vi "Automatic Frequency Linearization.vi"() -> ()   [LabVIEW 2014]
panel:
  out "Triangular skewtri generated from min factor":dbl[](graph)
  in  "Sample /Modulation Frequency":enum32{"40MHz/32KHz", "30MHz/24Khz"}(radio)=enum."30MHz/24Khz"
  in  "Scaling factor":dbl=1.0
  out "Rising Min Factor":dbl
  out "Falling Min Factor":dbl
  out "Rising Min DevStd%":dbl
  out "Falling Min DevStd%":dbl
  out "Fine?":bool
  out "Ok?":bool
  in  "#MeanMeasuraments":i32=50
  in  "StopValue":dbl=0.2
  in  "stop":bool
  out "Mean  FREQUENCY Curve Falling":dbl[](graph)
  out "Mean FREQUENCY Curve Rising":dbl[](graph)
  out "Current Skew Tri":dbl[](graph)
  out "Current Mul factor":dbl
  out "Current iteration (Countdown)":dbl
  out "Rising<= 1%":bool
  out "Falling<= 1%":bool
  in  "DeltaFactor":dbl=0.01
  in  "Initial Factor Mul":dbl=0.35
  out "2) Rising StdDev % Graph":cluster{dbl[], dbl[]}(graph)
  out "1) Falling StdDev % Graph":cluster{dbl[], dbl[]}(graph)
  out "2) Rising Std Dev %":dbl
  out "1) Falling Std Dev %":dbl
  out "2) Rising Signal (Last)":dbl[](graph)
  out "1) Falling Signal (Last)":dbl[](graph)
  in  "#LinMesuraments":i32=20
  # "OFFLINE SETUP"
  # "CURRENT ITERATION"
  # "Fattore moltiplicativo"
  # "Numero di misure su cui calcolare la curva delle frequenze medie con triangolo dritto"
  # "Numero di misurazioni\n su cui mediare durante la\nlinearizzazione"
  # "Optimal Factor Rising: 0.33    with Falling curve: 0.294"
  # "Optimal Factor Falling: 0.22/0.23"
  # "Fattore moltiplicativo\nIniziale"
  # "Passo del fattore\nmoltiplicativo"
  # "Fattore moltiplicativo\nFinale"
  # "%"
  # "%"
  # "FINAL RESULTS"
  # "Andamento della deviazione standard percentuale in funzione del fattore moltiplicativo"
  # "%"
  # "%"
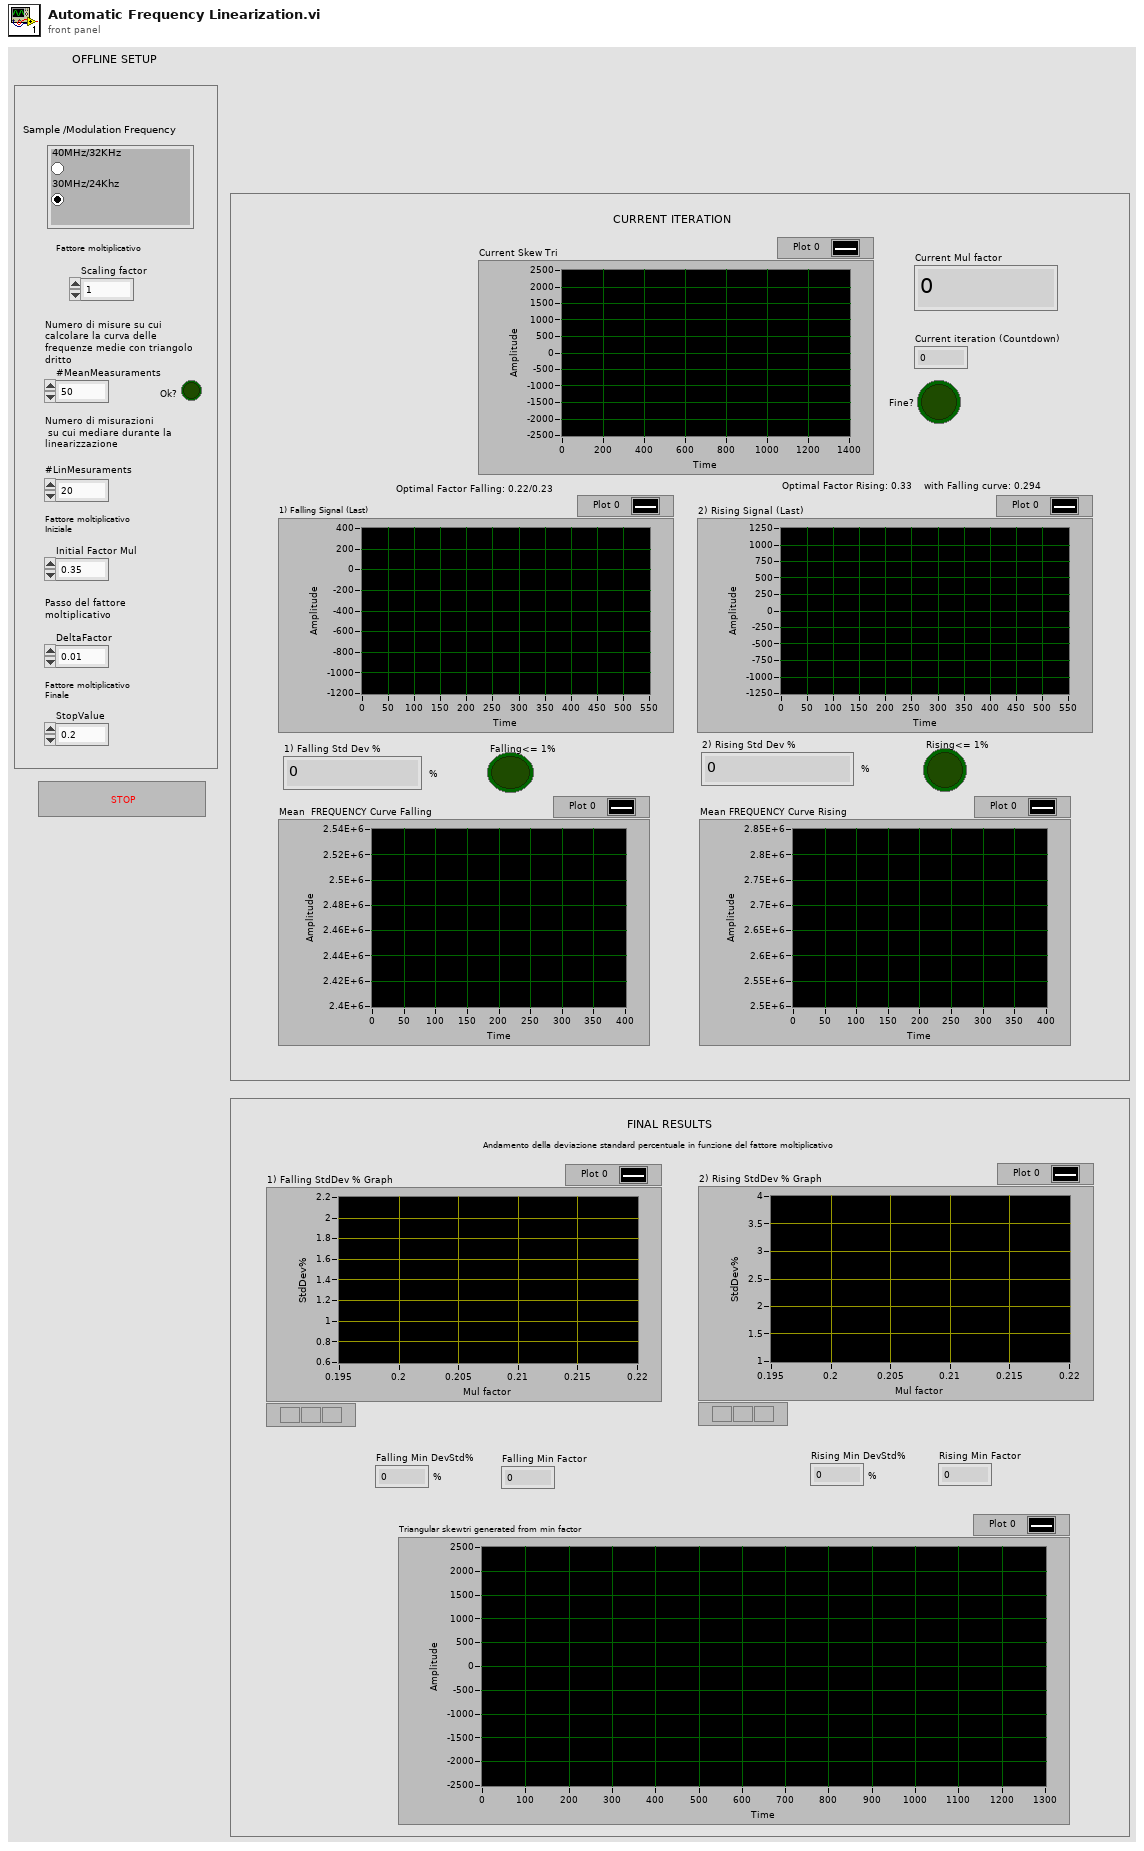
[diagram p1: front panel]
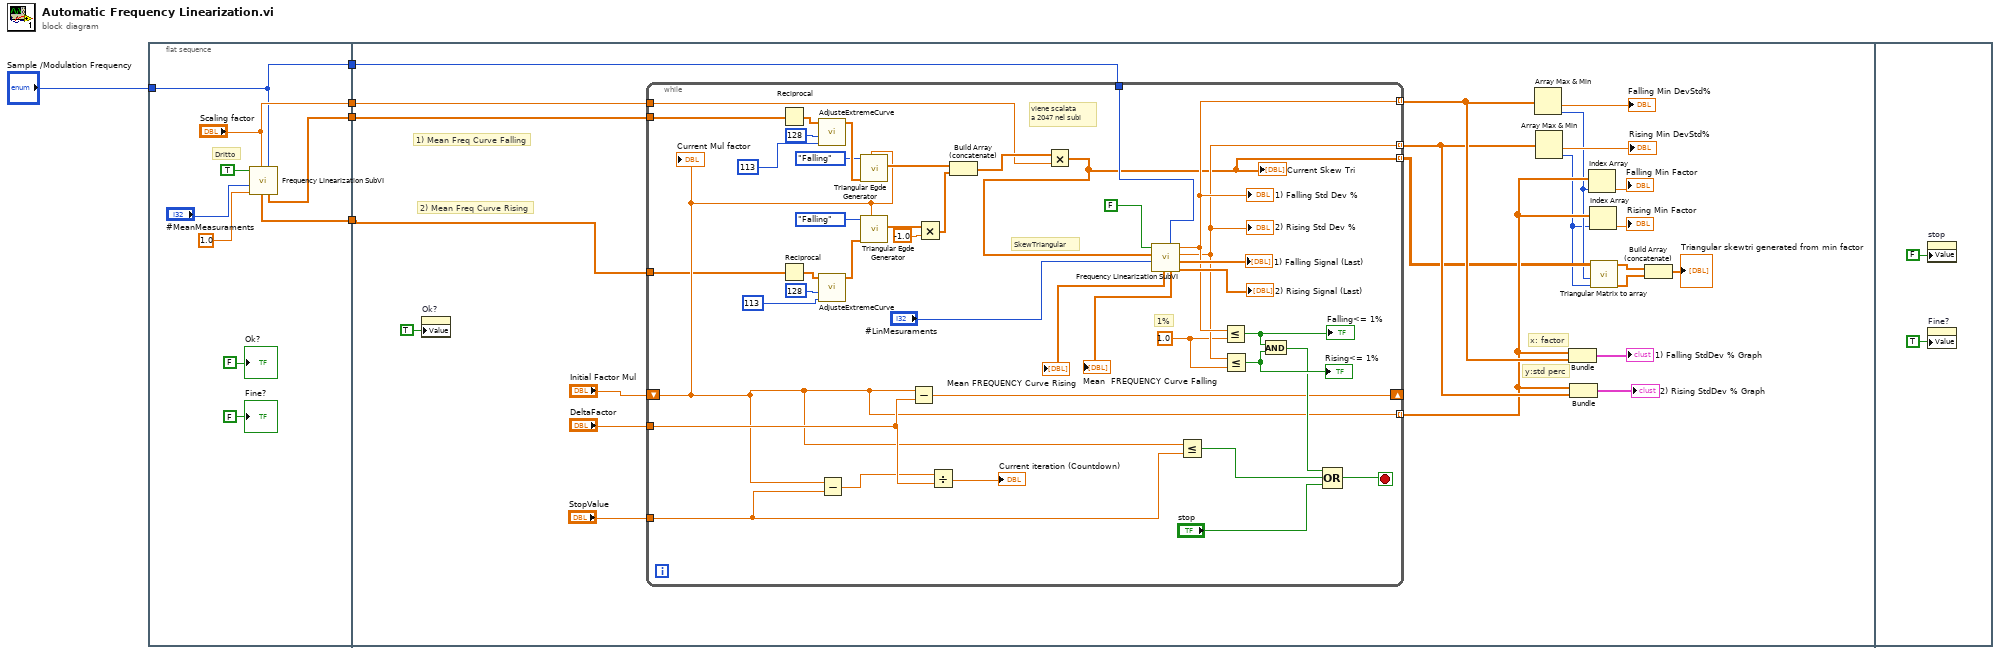
[diagram p0: block diagram]
diagram:
  n1 = flat-sequence {
    tunnel: [w12] -> w5
    tunnel: [w11] -> w4
    tunnel: ["Scaling factor"] -> w3
    tunnel: "Sample /Modulation Frequency" -> [w6]
    tunnel: [w6] -> w1
    tunnel: w5 -> [w23]
    tunnel: w4 -> [w24]
    tunnel: w3 -> [w22]
    tunnel: w1 -> [w21]
    frame #0 {
      # "Dritto"
      n2 = call "Frequency Linearization SubVI.vi"("Sample /Modulation Frequency"=w6, "Scaling factor"="Scaling factor", "Scale factor"=1.0, "#Medie"="#MeanMeasuraments", "Triangolo dritto"=TRUE) -> ("Last Mean Freq Curve Falling"=w12:dbl[], "Last Mean Freq Curve Rising"=w11:dbl[])  [unwired: 1 in, 4 out]
      "Ok?" <- FALSE ("Ok?")
      "Fine?" <- FALSE ("Ok?")
    }
    frame #1 {
      # "2) Mean Freq Curve Rising"
      # "1) Mean Freq Curve Falling"
      # "y:std perc"
      # "x: factor"
      n3 = property on="Ok?" class="Bool (strict)"("Value"=TRUE ("Ok?")) -> ()  [unwired: 2 in, 2 out]
      n4 = while {
        tunnel: [w74] -> w31 mode=indexing
        tunnel: [w73] -> w28 mode=indexing
        shift-right: [w49] -> _
        shift-left: "Initial Factor Mul" -> [w46]
        tunnel: "DeltaFactor" -> [w47]
        tunnel: w23 -> [w41]
        tunnel: w24 -> [w40]
        tunnel: [w46] -> w27 mode=indexing
        tunnel: "StopValue" -> [w45]
        tunnel: w22 -> [w42]
        tunnel: w21 -> [w39]
        tunnel: [w38] -> w20 mode=indexing
        stop <- w52 stop-if-true
        w72 = 1.0 ("y")
        # "viene scalata \na 2047 nel subi"
        # "SkewTriangular"
        # "1%"
        n5 = Reciprocal(x=w41) -> (1/x=w59:dbl[])
        n6 = Reciprocal(x=w40) -> (1/x=w70:dbl[])
        n7 = call "AdjusteExtremeCurve.vi"("Init Bins Discarded"=u32 113, "FFT Size Window"=128, "Freq sample"=w59) -> ("Extended Freq Sample"=w63:dbl[])  [unwired: 8 in]
        n8 = call "AdjusteExtremeCurve.vi"("Init Bins Discarded"=u32 113, "FFT Size Window"=128, "Freq sample"=w70) -> ("Extended Freq Sample"=w64:dbl[])  [unwired: 8 in]
        n9 = Subtract(x=w46, y=w45) -> (x-y=w44:dbl)
        n10 = call "Triangular Egde Generator.vi"("fattore"=w46, "Sample values"=w63, "Triangular edge"=enum16{"Rising", "Falling"}."Falling") -> ("Skew Triangular"=w62:dbl[])  [unwired: 8 in]
        n11 = call "Triangular Egde Generator.vi"("fattore"=w46, "Sample values"=w64, "Triangular edge"=enum16{"Rising", "Falling"}."Falling") -> ("Skew Triangular"=w66:dbl[])  [unwired: 8 in]
        n12 = Subtract(x=w46, y=w47) -> (x-y=w49:dbl)
        n13 = Multiply(x=w66, y=-1.0) -> (x*y=w67:dbl[])
        n14 = Divide(x=w44, y=w47) -> (x/y=→"Current iteration (Countdown)":dbl)
        n15 = Build Array (concatenate)(w62, w67) -> (w43:dbl[])
        n16 = Multiply(x=w43, y=w42) -> (x*y=w38:dbl[])
        "Current Skew Tri" <- w38
        n17 = call "Frequency Linearization SubVI.vi"("Sample /Modulation Frequency"=w39, "#Medie"="#LinMesuraments", "Sketri Input"=w38, "Triangolo dritto"=FALSE) -> ("Second Signal (Last)"=→"2) Rising Signal (Last)":dbl[], "First Signal (Last)"=→"1) Falling Signal (Last)":dbl[], "Rising Std Dev %"=w73:dbl, "Falling Std Dev %"=w74:dbl, "Last Mean Freq Curve Falling"=→"Mean  FREQUENCY Curve Falling":dbl[], "Last Mean Freq Curve Rising"=→"Mean FREQUENCY Curve Rising":dbl[])  [unwired: 2 in]
        "1) Falling Std Dev %" <- w74
        "2) Rising Std Dev %" <- w73
        n18 = Less Or Equal?(x=w46, y=w45) -> (x <= y?=w48:bool)
        n19 = Less Or Equal?(x=w74, y=w72) -> (x <= y?=w75:bool)
        "Falling<= 1%" <- w75
        n20 = Less Or Equal?(x=w73, y=w72) -> (x <= y?=w71:bool)
        "Rising<= 1%" <- w71
        n21 = And(x=w75, y=w71) -> (x .and. y?=w51:bool)
        n22 = Compound Arithmetic op=OR(w51, w48, "stop") -> (w52:bool)
        "Current Mul factor" <- w46
      }
      n23 = Array Max & Min(array=w31) -> (min value=→"Falling Min DevStd%":dbl, min index (indices)=w19:i32)  [unwired: 2 out]
      n24 = Array Max & Min(array=w28) -> (min value=→"Rising Min DevStd%":dbl, min index (indices)=w18:i32)  [unwired: 2 out]
      n25 = Bundle(w27, w31) -> (→"1) Falling StdDev % Graph":cluster{dbl[], dbl[]})  [unwired: 1 in]
      n26 = Bundle(w27, w28) -> (→"2) Rising StdDev % Graph":cluster{dbl[], dbl[]})  [unwired: 1 in]
      n27 = Index Array(array=w27, index=w19) -> (element=→"Falling Min Factor":dbl)
      n28 = Index Array(array=w27, index=w18) -> (element=→"Rising Min Factor":dbl)
      n29 = call "Triangular Matrix to array.vi"("index second subarray"=w18, "index first subarray"=w19, "Array"=w20) -> ("Array second"=w16:dbl[], "Array first"=w17:dbl[])  [unwired: 7 in]
      n30 = Build Array (concatenate)(w17, w16) -> (→"Triangular skewtri generated from min factor":dbl[])
    }
    frame #2 {
      n31 = property on="stop" class="Bool (strict)"("Value"=FALSE ("stop")) -> ()  [unwired: 2 in, 2 out]
      n32 = property on="Fine?" class="Bool (strict)"("Value"=TRUE ("Fine?")) -> ()  [unwired: 2 in, 2 out]
    }
  }
